vi "SCPI Decode.vi"(5 "Command String":string) -> (4 "Command [VERB]":string, 8 "Arguments [NOUNS]":string[](array[string]))   [LabVIEW 2016, in "SCPI.lvclass"]
uses:
  SCPI.lvclass
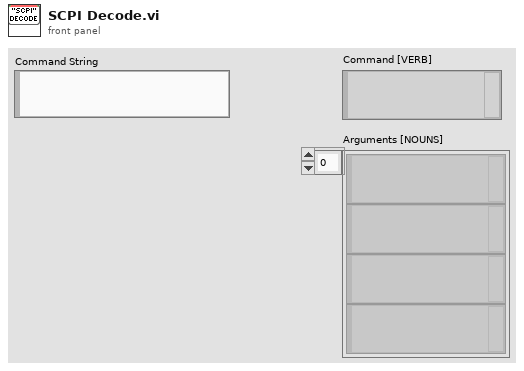
[diagram p1: front panel]
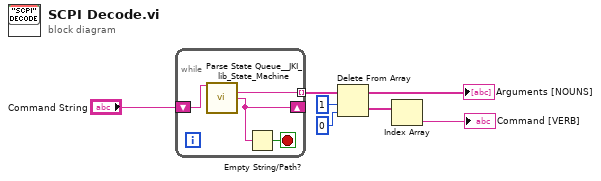
[diagram p0: block diagram]
diagram:
  n1 = while {
    tunnel: [w11] -> w7 mode=indexing
    shift-right: [w9] -> _
    shift-left: "Command String" -> [w10]
    stop <- w8 stop-if-true
    n2 = call <vilib>:"Parse State Queue__JKI_lib_State_Machine.vi"("State Queue"=w10) -> ("Current State"=w11:string, "Arguments"=w9:string)  [unwired: 12 in, 1 out]
    n3 = Empty String/Path?(string/path=w9) -> (empty?=w8:bool)
  }
  n4 = Delete From Array(array=w7, length=1, index=0) -> (deleted portion=w5:string[], array with subset deleted=→"Arguments [NOUNS]":string[])
  n5 = Index Array(array=w5) -> (element=→"Command [VERB]":string)  [unwired: 1 in]
